vi "test_232_imu-3d_MW-AHRSv1.vi"() -> ()   [LabVIEW 2019]
uses:
  Ctrl/cmd_common.ctl
  <vilib>/picture/3D Picture Control/Object/Create Object (name).vi
  <vilib>/Instr/_visa.llb/VISA Configure Serial Port (Instr).vi
  <vilib>/picture/3D Picture Control/NI_3D Picture Control.lvlib
panel:
  in  "탭 컨트롤":enum32{"cfg", "3d ui", "etc"}(tab)
  in  "Pitch":dbl(knob) scale=0.0..360.0
  in  "Roll":dbl(knob) scale=0.0..360.0
  in  "Yaw":dbl(knob) scale=0.0..360.0
  in  "w-data":string="ang"
  in  "Port":refnum<visa-resource-name>="COM24"
  in  "baud rate":u32=115200 caption="rate"
  out "3D Picture":refnum<vi>(3d-picture)
  out "Scene Display":refnum<vi>(3d-picture)
  out "error out":errorcluster caption="에러 출력"
  in  "w":bool
  out "r buff":u32(graph)
  in  "정지":bool
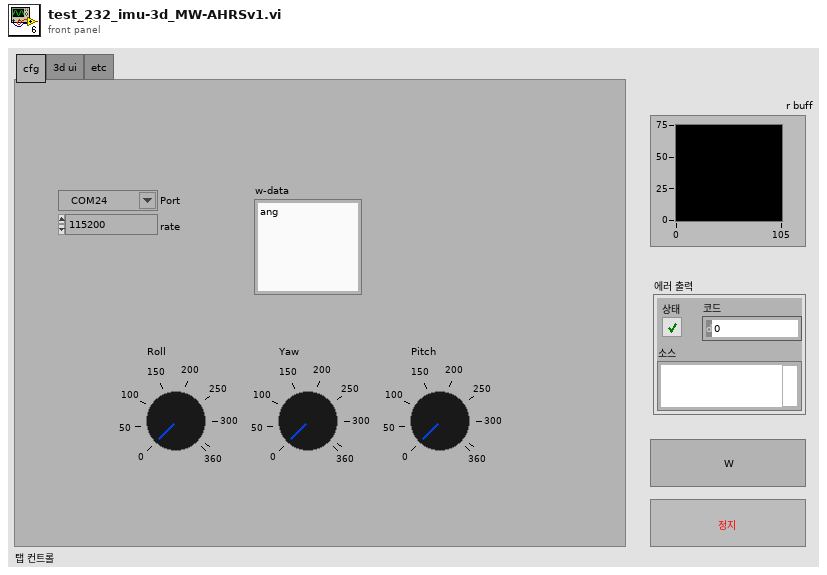
[diagram p1: front panel]
types:
  T1 = typedef "cmd_common.ctl" = enum16{"read", "write"}
  T2 = cluster{"angle":dbl[], "acc":dbl[], "mag":dbl[], "gyr":dbl[]}
  T3 = cluster{"angle[0]":dbl, "angle[1]":dbl, "angle[2]":dbl}
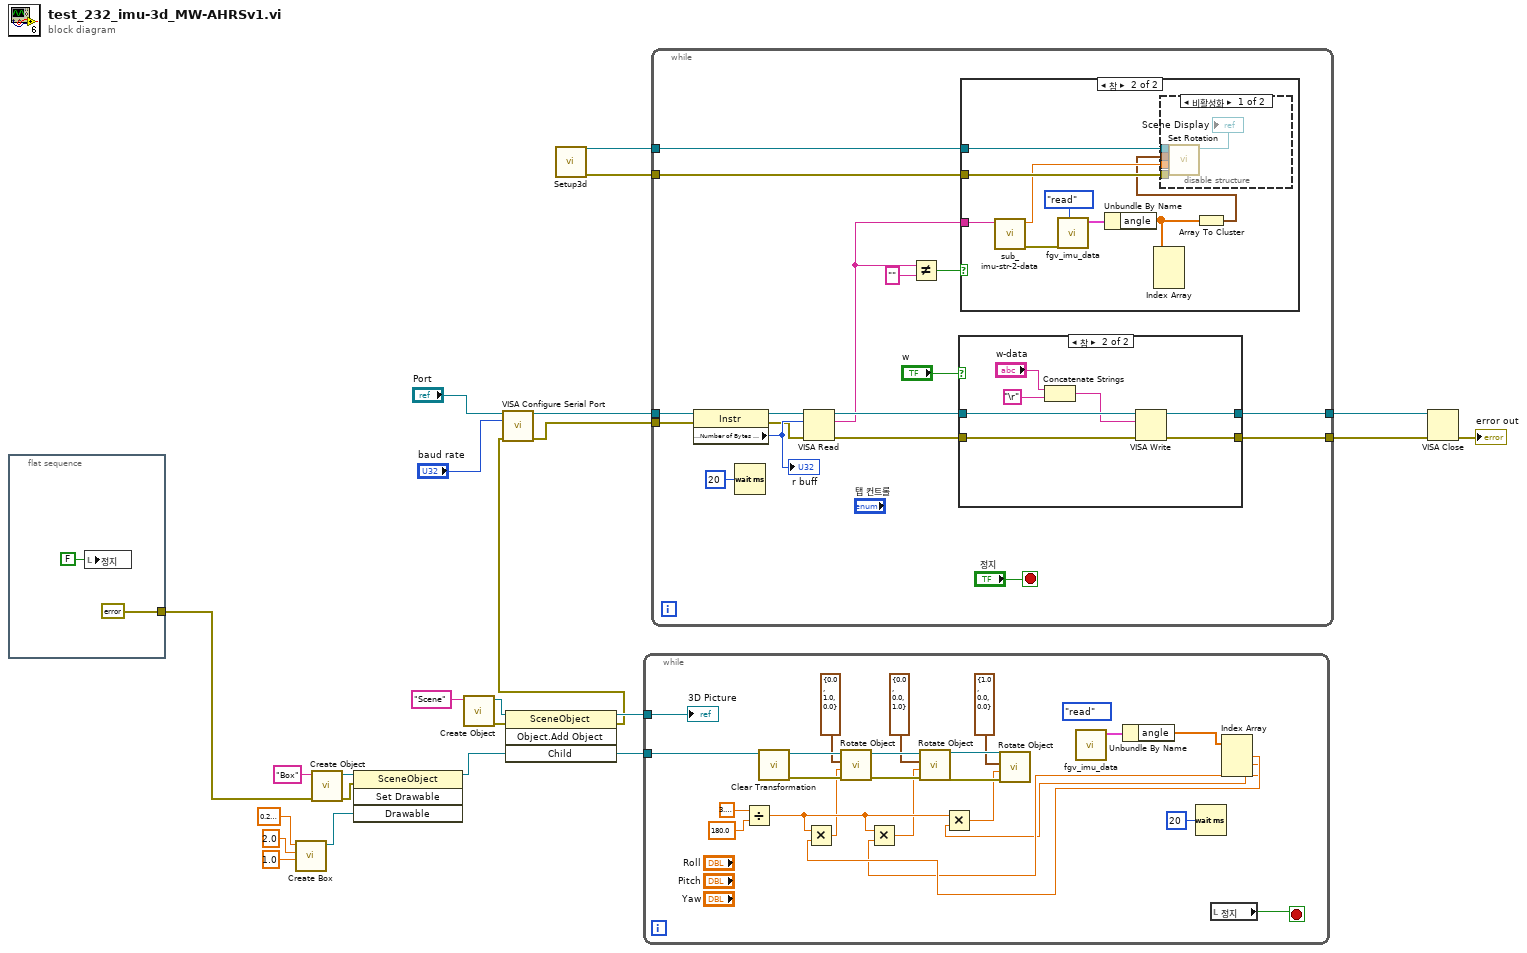
[diagram p0: block diagram]
diagram:
  n1 = flat-sequence {
    tunnel: [errorcluster {"status"=FALSE, "code"=0, "source"=""} ("error in (no error)")] -> w1
    frame #0 {
      n2 = local write "정지"(FALSE ("정지")) -> ()
    }
  }
  n3 = call <vilib>:"Create Box.vi"("Length Z"=sgl 1.0, "Length Y"=sgl 2.0, "Length X"=sgl 0.2) -> ("New Box Refnum"=w11:refnum<vi>)  [unwired: 7 in, 1 out]
  n4 = call-poly <vilib>:"Create Object.vi"("error in (no error)"=w1, "Name"="Box") -> ("error out"=w10:errorcluster, "Scene:New Object"=w9:refnum<vi>)  [unwired: 8 in]
  n5 = invoke class="SceneObject" method="Set Drawable"(reference=w9, error in=w10, "Drawable"=w11) -> (reference out=w15:refnum<vi>)  [unwired: 1 in, 3 out]
  n6 = call-poly <vilib>:"Create Object.vi"("Name"="Scene") -> ("error out"=w14:errorcluster, "Scene:New Object"=w13:refnum<vi>)  [unwired: 9 in]
  n7 = invoke class="SceneObject" method="Object.Add Object"(reference=w13, error in=w14, "Child"=w15) -> (reference out=w4:refnum<vi>, error out=w2:errorcluster, "Child"=w3:refnum<vi>)  [unwired: 1 in, 1 out]
  n8 = call-poly "VISA Configure Serial Port"("VISA resource name"="Port", "baud rate (9600)"="baud rate", "error in (no error)"=w2) -> ("VISA resource name out"=w19:refnum<visa-resource-name>, "error out"=w20:errorcluster)  [unwired: 11 in]
  n9 = call "Setup3d.vi"() -> ("error out"=w24:errorcluster, "Scene Object"=w23:refnum<vi>)  [unwired: 10 in]
  n10 = while {
    tunnel: w4 -> [w36]
    tunnel: w3 -> [w50]
    stop <- w33 stop-if-true
    (unwired) cmd_common."read" ("cmd")
    n11 = Divide(x=3.141592653589793, y=180.0) -> (x/y=w38:dbl)
    n12 = call <vilib>:"Clear Transformation.vi"("Object Refnum In"=w50) -> ("error out"=w46:errorcluster, "Object Refnum Out"=w47:refnum<vi>)  [unwired: 9 in]
    n13 = call "fgv_imu_data.vi"() -> ("IMD data out"=w31:T2)  [unwired: 10 in, 1 out]
    n14 = Unbundle By Name(w31) -> ("angle"=w30:dbl[])
    n15 = Wait (ms)(milliseconds to wait=u32 20 ("대기 시간 (ms)")) -> ()  [unwired: 1 out]
    n16 = local read "정지"() -> (w33:bool)
    n17 = Index Array(array=w30) -> (element #1=w29:dbl, element #2=w28:dbl, element #3=w27:dbl)  [unwired: 3 in]
    n18 = Multiply(x=w38, y=w29) -> (x*y=w35:dbl)
    n19 = call <vilib>:"Rotate Object.vi"("error in (no error)"=w46, "Angle"=w35, "Axis"=cluster{"X":sgl, "Y":sgl, "Z":sgl} {"X"=0.0, "Y"=1.0, "Z"=0.0}, "Scene.Object In"=w47) -> ("error out"=w48:errorcluster, "Scene.Object Out"=w49:refnum<vi>)  [unwired: 6 in]
    n20 = Multiply(x=w38, y=w28) -> (x*y=w34:dbl)
    n21 = call <vilib>:"Rotate Object.vi"("error in (no error)"=w48, "Angle"=w34, "Axis"=cluster{"X":sgl, "Y":sgl, "Z":sgl} {"X"=0.0, "Y"=0.0, "Z"=1.0}, "Scene.Object In"=w49) -> ("error out"=w41:errorcluster, "Scene.Object Out"=w42:refnum<vi>)  [unwired: 6 in]
    n22 = Multiply(x=w38, y=w27) -> (x*y=w37:dbl)
    n23 = call <vilib>:"Rotate Object.vi"("error in (no error)"=w41, "Angle"=w37, "Axis"=cluster{"X":sgl, "Y":sgl, "Z":sgl} {"X"=1.0, "Y"=0.0, "Z"=0.0}, "Scene.Object In"=w42) -> ()  [unwired: 6 in, 2 out]
    "3D Picture" <- w36
  }
  n24 = while {
    tunnel: w24 -> [w52]
    tunnel: w23 -> [w51]
    tunnel: w20 -> [w62]
    tunnel: w19 -> [w61]
    tunnel: [w57] -> w17
    tunnel: [w56] -> w16
    stop <- "정지" stop-if-true
    n25 = property class="Instr"(reference=w61, error in=w62) -> (reference out=w66:refnum<visa-resource-name>, error out=w63:errorcluster, "Serial Settings:Number of Bytes at Serial Port"=w64:u32)
    "r buff" <- w64
    n26 = Wait (ms)(milliseconds to wait=u32 20 ("대기 시간 (ms)")) -> ()  [unwired: 1 out]
    n27 = VISA Read(VISA resource name=w66, byte count=w64, error in (no error)=w63) -> (VISA resource name out=w58:refnum<visa-resource-name>, read buffer=w53:string, error out=w59:errorcluster)  [unwired: 1 out]
    n28 = Not Equal?(x=w53, y="") -> (x != y?=w55:bool)
    n29 = case shown="참" "w" {
      tunnel: w58 -> [w83 w90]
      tunnel: [w83 w89] -> w57
      tunnel: w59 -> [w82 w88]
      tunnel: [w82 w87] -> w56
      frame False {
      }
      frame True {
        n30 = Concatenate Strings("w-data", "\r") -> (w84:string)
        n31 = VISA Write(VISA resource name=w90, write buffer=w84, error in (no error)=w88) -> (VISA resource name out=w89:refnum<visa-resource-name>, error out=w87:errorcluster)  [unwired: 1 out]
      }
    }
    n32 = case shown="참" w55 {
      tunnel: w53 -> [_ w76]
      tunnel: w52 -> [_ w75]
      tunnel: w51 -> [_ w74]
      frame False {
      }
      frame True {
        n33 = call "sub_imu-str-2-data.vi"("read buffer"=w76) -> ("error out"=w72:errorcluster, "heading"=w70:dbl)  [unwired: 9 in]
        n34 = call "fgv_imu_data.vi"("cmd"=cmd_common."read", "error in"=w72) -> ("IMD data out"=w71:T2)  [unwired: 8 in, 1 out]
        n35 = Unbundle By Name(w71) -> ("angle"=w69:dbl[])
        n36 = Index Array(array=w69) -> ()  [unwired: 3 in, 3 out]
        n37 = Array To Cluster(array=w69) -> (cluster=w68:T3)
        n38 = disable-structure shown="비활성화" {
          disable-tunnel: w75 -> [w80 _]
          disable-tunnel: w74 -> [w79 _]
          disable-tunnel: w70 -> [w78 _]
          disable-tunnel: w68 -> [w77 _]
          frame Disabled {
            n39 = call <vilib>:"Set Rotation.vi"("error in (no error)"=w80, "Angle"=w78, "Axis"=w77, "Scene Object"=w79) -> ("Rotated Scene Object"=→"Scene Display":refnum<vi>)  [unwired: 6 in, 1 out]
          }
          frame Enabled {
          }
        }
      }
    }
  }
  n40 = VISA Close(VISA resource name=w17, error in (no error)=w16) -> (error out=→"error out":errorcluster)
